vi "directory_structure_creator.vi"(1 "Path to be created":path) -> (0 "Duplicate \"Path to be created\"":path)   [LabVIEW 2017]
doc: "This VI demonstrates how to create a directory within a directory when the higher-level directory does not yet exist. This VI uses the Queue Operations to create each directory needed to complete the hierarchy specified by the path you enter."
panel:
  # "Directions:\n\n1. Enter the path to the directory you want to create in the Path to be created field.\n2. Run the VI. LabVIEW creates the new directory and any higher level directories that did not previously exist.\n\nSelect Help»Show Context Help and move the cursor over the VI icon to display help for this VI."
  # "Purpose:\n\nCurrently the New Directory VI on the Advanced File Functions palette can create a directory only in a directory that already exists. If you want to create C:\\a\\b\\c, but only C:\\a exists, LabVIEW returns an error. This VI uses the Queue Operation to build the directory structure you specify in the \"Path to be created\" control regardless of the current structure. You can create C:\\a\\b\\c in a single step even if only C:\\a exists."
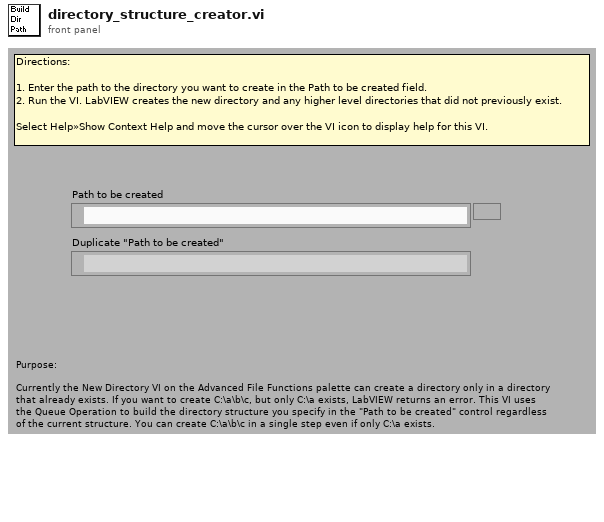
[diagram p1: front panel]
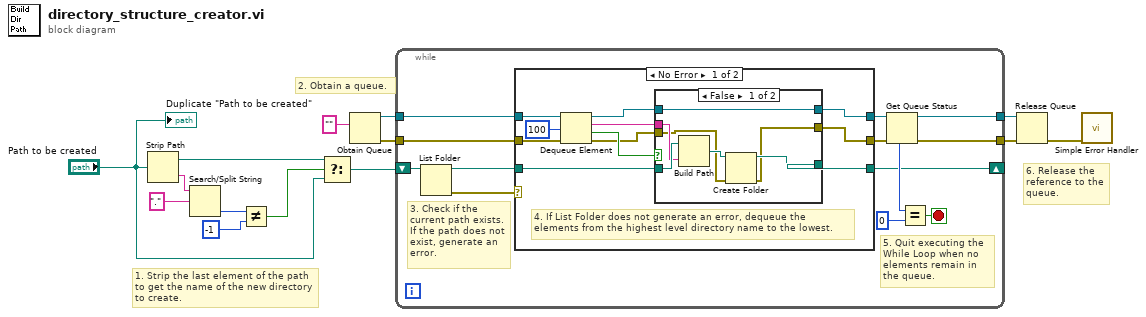
[diagram p0: block diagram]
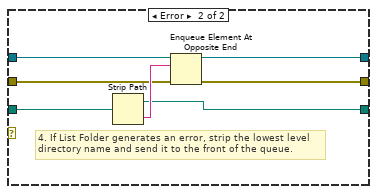
[diagram p3: hidden frame]
diagram:
  # "2. Obtain a queue."
  # "6. Release the reference to the queue."
  # "1. Strip the last element of the path to get the name of the new directory to create."
  n1 = Strip Path(path="Path to be created") -> (stripped path=w5:path, name=w11:string)
  n2 = Search/Split String(string=w11, search string/char (-)="." ("regular expression")) -> (offset of match=w2:i32)  [unwired: 1 in, 2 out]
  n3 = Not Equal?(x=w2, y=-1) -> (x != y?=w3:bool)
  n4 = Select(t=w5, s=w3, f="Path to be created") -> (s? t:f=w4:path)
  n5 = Obtain Queue(element data type="") -> (queue out=w14:refnum<queue>, error out=w9:errorcluster)  [unwired: 4 in, 1 out]
  n6 = while {
    shift-right: [w19] -> _
    shift-left: w4 -> [w26]
    tunnel: w14 -> [w27]
    tunnel: [w23] -> w13
    tunnel: w9 -> [w18]
    tunnel: [w16] -> w8
    stop <- w22 stop-if-true
    # "5. Quit executing the While Loop when no elements remain in the queue."
    # "3. Check if the current path exists. If the path does not exist, generate an error."
    n7 = List Folder(path=w26) -> (path out=w25:path, error out=w15:errorcluster)  [unwired: 3 in, 2 out]
    n8 = case shown="No Error" w15 {
      tunnel: w27 -> [w35 w55]
      tunnel: [w32 w54] -> w24
      tunnel: w25 -> [w38 w52]
      tunnel: [w37 w51] -> w19
      tunnel: w18 -> [w31 w50]
      tunnel: [w29 w49] -> w17
      frame No Error {
        # "4. If List Folder does not generate an error, dequeue the elements from the highest level directory name to the lowest."
        n9 = Dequeue Element(queue=w35, timeout in ms (-1)=100, error in (no error)=w31) -> (queue out=w33:refnum<queue>, element=w36:string, timed out?=w34:bool, error out=w30:errorcluster)
        n10 = case shown="False" w34 {
          tunnel: w38 -> [w45 w48]
          tunnel: [w44 w48] -> w37
          tunnel: w36 -> [w43 _]
          tunnel: w33 -> [w41 w47]
          tunnel: [w41 w47] -> w32
          tunnel: w30 -> [w40 w46]
          tunnel: [w39 w46] -> w29
          frame False {
            n11 = Build Path(base path=w45, name or relative path=w43) -> (appended path=w42:path)
            n12 = Create Folder(path (use dialog)=w42, error in=w40) -> (created path=w44:path, error out=w39:errorcluster)  [unwired: 1 in, 1 out]
          }
          frame True {
          }
        }
      }
      frame Error {
        # "4. If List Folder generates an error, strip the lowest level directory name and send it to the front of the queue."
        n13 = Strip Path(path=w52) -> (stripped path=w51:path, name=w53:string)
        n14 = Enqueue Element At Opposite End(queue=w55, element=w53, error in (no error)=w50) -> (queue out=w54:refnum<queue>, error out=w49:errorcluster)  [unwired: 1 in, 1 out]
      }
    }
    n15 = Get Queue Status(queue=w24, error in (no error)=w17) -> (queue out=w23:refnum<queue>, error out=w16:errorcluster, # elements in queue=w21:i32)  [unwired: 1 in, 5 out]
    n16 = Equal?(x=w21, y=0) -> (x = y?=w22:bool)
  }
  n17 = Release Queue(queue=w13, error in (no error)=w8) -> (error out=w7:errorcluster)  [unwired: 1 in, 2 out]
  n18 = call <vilib>:"Simple Error Handler.vi"("error in (no error)"=w7) -> ()  [unwired: 4 in, 5 out]
  "Duplicate \"Path to be created\"" <- "Path to be created"
